vi "Teleop.vi"(10 "Match Info":T2={"Autonomous Elapsed Seconds"=0.0, "TeleOp Elapsed Seconds"=0.0, "Disabled Elapsed Seconds"=0.0, "Visited Autonomous"=FALSE, "Visited TeleOp"=FALSE, "Visited Disabled"=FALSE, "Autonomous Settings"={"Autonomous Style"=enum."Independent", "VI Refnum"=refnum}}, 11 "Call Context":T3) -> ()   [LabVIEW 2019]
doc: "This VI is called for each TeleOp packet received from the DS where the robot is not disabled. It is often used to read from the joysticks and update I/O or to update setpoints for timed control loops. It should complete and return within 20 milliseconds or it may miss DS packets."
uses:
  <vilib>/Rock Robotics/WPI/DriverStation/WPI_DriverStationDerivedRobotMode.ctl
  <vilib>/Rock Robotics/WPI/DriverStation/WPI_DriverStationMatch Info.ctl
  <vilib>/Rock Robotics/WPI/ThirdParty/Phoenix-LabVIEW/Motor Controller/Controls/CTRE_Phoenix_MotorControl_ControlMode.ctl
  <vilib>/Rock Robotics/WPI/Solenoid/WPI_SolenoidValue.ctl
  <vilib>/Rock Robotics/Network Tables/NT Read Boolean.vi
  <vilib>/Rock Robotics/Network Tables/NT Read Number.vi
  <vilib>/Rock Robotics/WPI/Utilities/WPI_GetSetVariantRefNum.vi
  Robot Global Data.vi
  <vilib>/addons/control/pid/pid.llb/PID (DBL).vi
  <vilib>/Rock Robotics/Network Tables/NT Write Number.vi
  <vilib>/Rock Robotics/Network Tables/NT Write Numeric Array.vi
  <vilib>/Rock Robotics/WPI/Solenoid/WPI_SolenoidSetEnum.vi
  <vilib>/addons/control/pid/NI_PID_pid.lvlib
  <vilib>/Rock Robotics/Network Tables/NT Write Boolean.vi
  <vilib>/Rock Robotics/Network Tables/NT Write Boolean Array.vi
  <vilib>/Rock Robotics/Network Tables/NT Write String.vi
panel:
  in  "PID gains":T1={"proportional gain (Kc)"=1.0, "integral time (Ti, min)"=0.01, "derivative time (Td, min)"=0.0} {"derivative time (Td, min)" format="%.3f"; "integral time (Ti, min)" format="%.3f"; "proportional gain (Kc)" format="%.3f"}
  out "Sample Slider 0":dbl(slide) scale=0.0..5.0
  out "Sample Boolean 1":bool
  out "Sample Boolean 0":bool
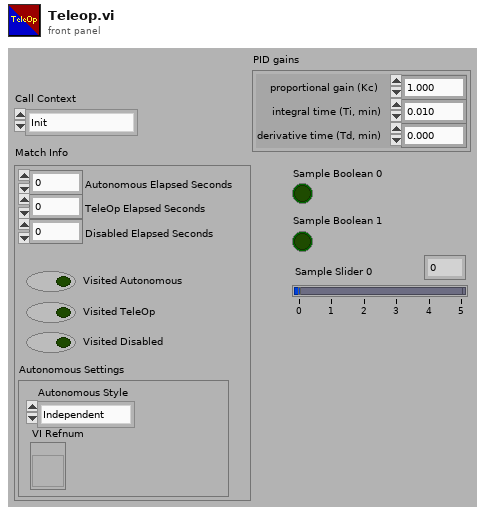
[diagram p1: front panel]
types:
  T1 = cluster{"proportional gain (Kc)":dbl, "integral time (Ti, min)":dbl, "derivative time (Td, min)":dbl}
  T2 = typedef "WPI_DriverStationMatch Info.ctl" = cluster{"Autonomous Elapsed Seconds":dbl, "TeleOp Elapsed Seconds":dbl, "Disabled Elapsed Seconds":dbl, "Visited Autonomous":bool, "Visited TeleOp":bool, "Visited Disabled":bool, "Autonomous Settings":cluster{"Autonomous Style":enum16{"Iterative", "Independent"}, "VI Refnum":refnum<vi>}}
  T3 = typedef "WPI_DriverStationDerivedRobotMode.ctl" = enum16{"Init", "Execute", "Stop"}
  T4 = typedef "CTRE_Phoenix_MotorControl_ControlMode.ctl" = u16
  T5 = typedef "WPI_JoystickDevRef.ctl" = cluster{"Device":T6}
  T6 = typedef "WPI_JoystickDeviceEnum.ctl" = enum16{"USB 0", "USB 1", "USB 2", "USB 3", "USB 4", "USB 5"}
  T7 = typedef "WPI_RobotDriveDevRef.ctl" = cluster{"DevStatus":errorcluster, "Motors[]":T8[], "Square Inputs":bool, "Max Output":dbl}
  T8 = typedef "WPI_MotorControlDeviceRef.ctl" = cluster{"DeviceStatus":errorcluster, "Type":T9, "PWM":cluster{"PWM Channel":T10, "DeadBand":T11}, "CAN":cluster{"Device Number":u8, "SetOutput VI Ref":variant, "GetOutput VI Ref":variant, "Enable VI Ref":variant, "Disable VI Ref":variant, "Data":variant}, "Invert":bool, "DIO PWM":cluster{"PWM \"Enable\" Channel":T10, "DIOChannel":T12, "PWM Rate":dbl}}
  T9 = typedef "WPI_MotorControlType.ctl" = enum16{"PWM", "CAN", "DIO PWM"}
  T10 = typedef "FPGA_DIOPWMChannel.ctl" = enum8{"PWM 0", "PWM 1", "PWM 2", "PWM 3", "PWM 4", "PWM 5", "PWM 6", "PWM 7", "PWM 8", "PWM 9", "PWM MXP 0", "PWM MXP 1", "PWM MXP 2", "PWM MXP 3", "PWM MXP 4", "PWM MXP 5", "PWM MXP 6", "PWM MXP 7", "PWM MXP 8", "PWM MXP 9", "Invalid"}
  T11 = typedef "WPI_PWMDeadband.ctl" = cluster{"Name":string, "maxPositivePwm":i32, "minPositivePwm":i32, "centerPwm":i32, "maxNegativePwm":i32, "minNegativePwm":i32, "angularRange":u16}
  T12 = typedef "FPGA_DIOChannel.ctl" = enum8{"DIO 0", "DIO 1", "DIO 2", "DIO 3", "DIO 4", "DIO 5", "DIO 6", "DIO 7", "DIO 8", "DIO 9", "DIO MXP 0", "DIO MXP 1", "DIO MXP 2", "DIO MXP 3", "DIO MXP 4", "DIO MXP 5", "DIO MXP 6", "DIO MXP 7", "DIO MXP 8", "DIO MXP 9", "DIO MXP 10", "DIO MXP 11", "DIO MXP 12", "DIO MXP 13", "DIO MXP 14", "DIO MXP 15", "SPI Port CS1", "SPI Port CS2", "SPI Port CS3", "SPI Port MISO", "SPI Port MOSI", "Invalid"}
  T13 = cluster{"Buttons[0]":bool, "Buttons[1]":bool, "Buttons[2]":bool, "Buttons[3]":bool, "Buttons[4]":bool, "Buttons[5]":bool, "Buttons[6]":bool, "Buttons[7]":bool, "Buttons[8]":bool, "Buttons[9]":bool}
  T14 = cluster{"Axes[0]":dbl, "Axes[1]":dbl, "Axes[2]":dbl, "Axes[3]":dbl, "Axes[4]":dbl, "Axes[5]":dbl, "Axes[6]":dbl, "Axes[7]":dbl, "Axes[8]":dbl}
  T15 = typedef "WPI_DriverStationAllianceInfo.ctl" = enum16{"Red", "Blue", "Invalid"}
  T16 = typedef "WPI_SolenoidDevRef.ctl" = cluster{"DevStatus":errorcluster, "Pneumatics Control Module":u8, "Forward Solenoid Channel":T17, "Reverse Solenoid Channel":T17}
  T17 = typedef "WPI_SolenoidChannel.ctl" = enum8{"Solenoid 0", "Solenoid 1", "Solenoid 2", "Solenoid 3", "Solenoid 4", "Solenoid 5", "Solenoid 6", "Solenoid 7", "Invalid"}
  T18 = typedef "WPI_SolenoidValue.ctl" = enum16{"Off", "On", "Forward", "Reverse"}
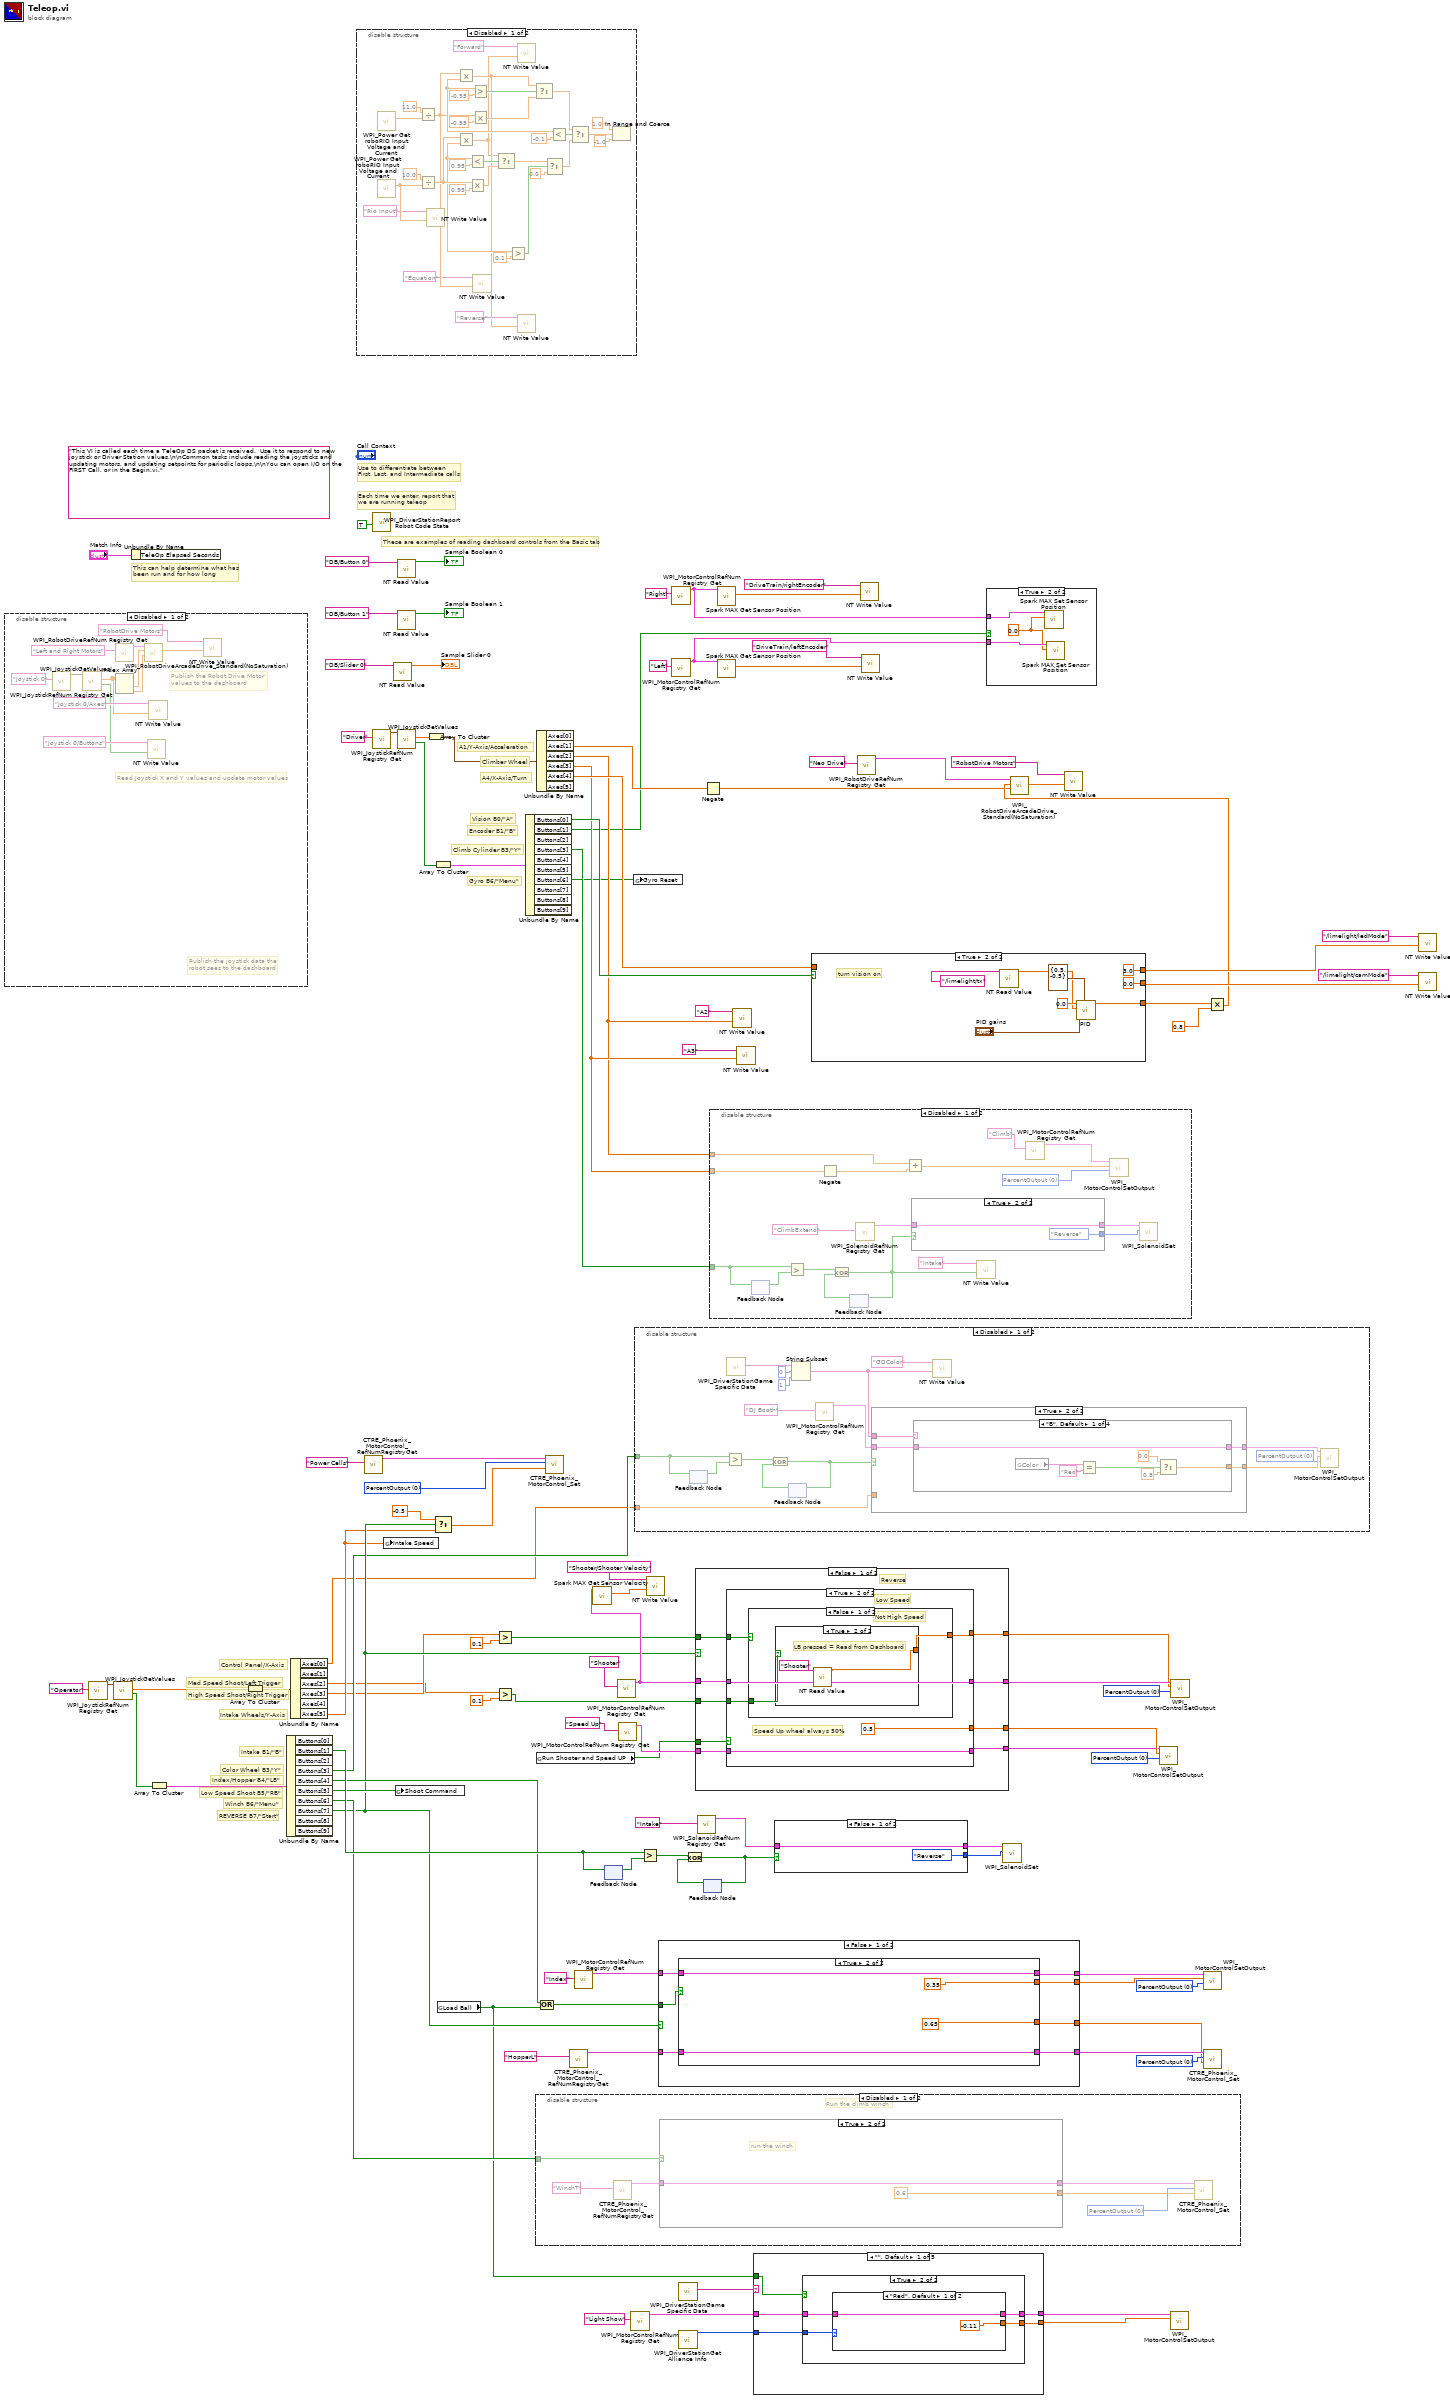
[diagram p0: block diagram]
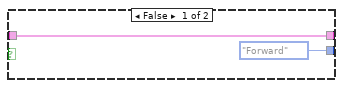
[diagram p2: hidden frame]
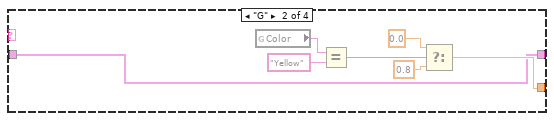
[diagram p5: hidden frame]
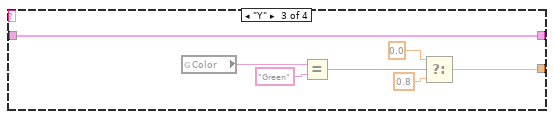
[diagram p6: hidden frame]
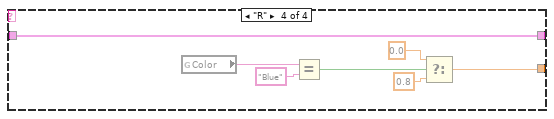
[diagram p7: hidden frame]
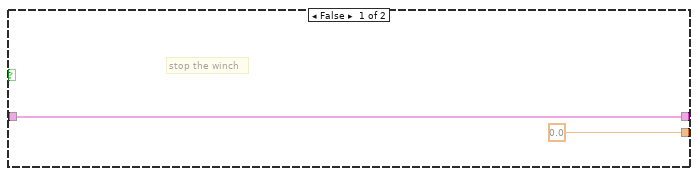
[diagram p9: hidden frame]
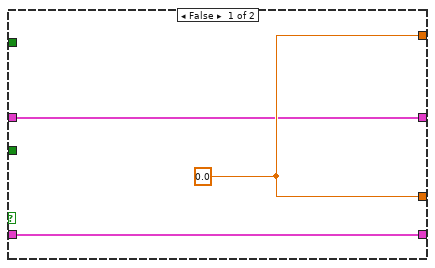
[diagram p12: hidden frame]
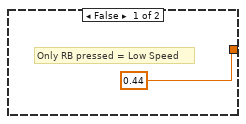
[diagram p13: hidden frame]
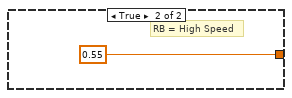
[diagram p14: hidden frame]
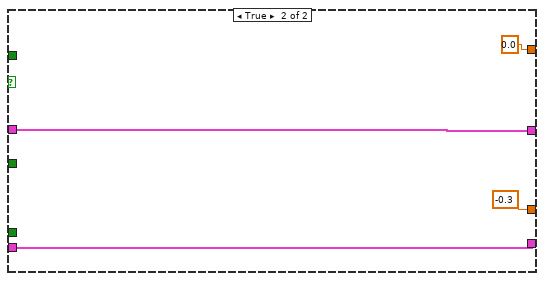
[diagram p15: hidden frame]
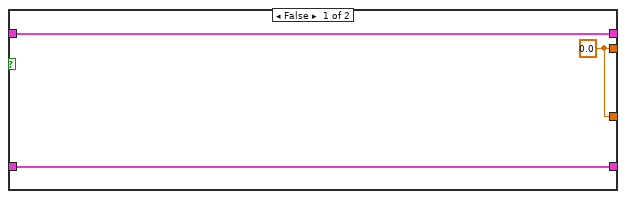
[diagram p16: hidden frame]
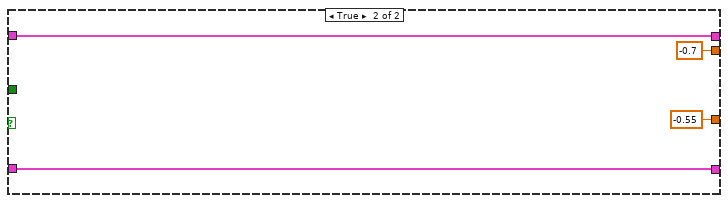
[diagram p17: hidden frame]
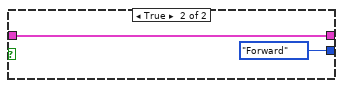
[diagram p18: hidden frame]
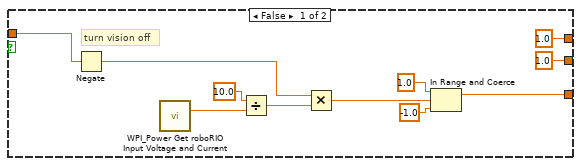
[diagram p20: hidden frame]
diagram:
  w46 = T4 0 items=["PercentOutput"=0, "Position"=1, "Velocity"=2, "Current"=3, "Follower"=5, "MotionProfile"=6, "MotionMagic"=7, "MotionProfileArc"=10, "Disabled"=15] ("Control Mode")
  w49 = T4 0 items=["PercentOutput"=0, "Position"=1, "Velocity"=2, "Current"=3, "Follower"=5, "MotionProfile"=6, "MotionMagic"=7, "MotionProfileArc"=10, "Disabled"=15] ("Control Mode")
  w56 = T4 0 items=["PercentOutput"=0, "Position"=1, "Velocity"=2, "Current"=3, "Follower"=5, "MotionProfile"=6, "MotionMagic"=7, "MotionProfileArc"=10, "Disabled"=15] ("Control Mode")
  w62 = T4 0 items=["PercentOutput"=0, "Position"=1, "Velocity"=2, "Current"=3, "Follower"=5, "MotionProfile"=6, "MotionMagic"=7, "MotionProfileArc"=10, "Disabled"=15] ("Control Mode")
  w64 = T4 0 items=["PercentOutput"=0, "Position"=1, "Velocity"=2, "Current"=3, "Follower"=5, "MotionProfile"=6, "MotionMagic"=7, "MotionProfileArc"=10, "Disabled"=15] ("Control Mode")
  (unwired) "This VI is called each time a TeleOp DS packet is received.  Use it to respond to new joystick or Driver Station values.\n\nCommon tasks include reading the joysticks and updating motors, and updating setpoints for periodic loops.\n\nYou can open I/O on the FIRST Call, or in the Begin.vi."
  # "Med Speed Shoot/Left Trigger"
  # "High Speed Shoot/Right Trigger"
  # "Color Wheel B3/'Y\""
  # "Gyro B6/\"Menu\""
  # "Encoder B1/\"B\""
  # "Climber Wheel"
  # "Climb Cylinder B3/\"Y\""
  # "A1/Y-Axis/Acceleration"
  # "A4/X-Axis/Turn"
  # "Vision B0/\"A\""
  # "Control Panel/X-Axis"
  # "Intake Wheels/Y-Axis"
  # "REVERSE B7/\"Start\""
  # "Winch B6/\"Menu\""
  # "Low Speed Shoot B5/\"RB\""
  # "Index/Hopper B4/\"LB\""
  # "Intake B1/\"B\""
  # "These are examples of reading dashboard controls from the Basic tab"
  # "Each time we enter, report that\nwe are running teleop"
  # "Use to differentiate between\nFirst, Last, and Intermediate calls"
  # "This can help determine what has\nbeen run and for how long"
  n1 = disable-structure shown="Disabled" {
    frame Disabled {
      # "Publish the Robot Drive Motor\nvalues to the dashboard"
      # "Publish the joystick data the\nrobot sees to the dashboard"
      # "Read Joystick X and Y values and update motor values"
      n2 = call <vilib>:"WPI_JoystickRefNum Registry Get.vi"("refnum name"="Joystick 0") -> ("JoystickDevRef"=w116:T5)  [unwired: 1 in, 9 out]
      n3 = call <vilib>:"WPI_JoystickGetValues.vi"("JoystickDevRef"=w116) -> ("Buttons"=w111:bool[], "Axes"=w112:dbl[])  [unwired: 6 in, 3 out]
      n4 = call <vilib>:"WPI_RobotDriveRefNum Registry Get.vi"("refnum name"="Left and Right Motors") -> ("RobotDriveDevRef"=w119:T7)  [unwired: 1 in, 9 out]
      n5 = Index Array(array=w112) -> (element #1=w118:dbl, element #2=w115:dbl)  [unwired: 2 in]
      n6 = call <vilib>:"WPI_RobotDriveArcadeDrive_Standard(NoSaturation).vi"("Y axis value"=w115, "X axis value"=w118, "RobotDriveDevRef"=w119) -> ("Motor Values"=w110:dbl[])  [unwired: 1 in, 7 out]
      n7 = call-poly <vilib>:"NT Write Value.vi"("Boolean Array"=w111, "Name"="Joystick 0/Buttons") -> ()  [unwired: 9 in, 1 out]
      n8 = call-poly <vilib>:"NT Write Value.vi"("Numeric Array"=w112, "Name"="Joystick 0/Axes") -> ()  [unwired: 9 in, 1 out]
      n9 = call-poly <vilib>:"NT Write Value.vi"("Numeric Array"=w110, "Name"="RobotDrive Motors") -> ()  [unwired: 9 in, 1 out]
    }
    frame Enabled {
    }
  }
  n10 = call <vilib>:"WPI_JoystickRefNum Registry Get.vi"("refnum name"="Operator") -> ("JoystickDevRef"=w75:T5)  [unwired: 9 in, 1 out]
  n11 = call <vilib>:"WPI_JoystickGetValues.vi"("JoystickDevRef"=w75) -> ("Buttons"=w48:bool[], "Axes"=w79:dbl[])  [unwired: 6 in, 3 out]
  n12 = Unbundle By Name("Match Info") -> ()  [unwired: 1 out]
  n13 = Array To Cluster(array=w48) -> (cluster=w77:T13)
  n14 = Array To Cluster(array=w79) -> (cluster=w78:T14)
  n15 = Unbundle By Name(w77) -> ("Buttons[1]"=w42:bool, "Buttons[3]"=w10:bool, "Buttons[4]"=w41:bool, "Buttons[5]"=w38:bool, "Buttons[6]"=w37:bool, "Buttons[7]"=w30:bool)  [unwired: 4 out]
  n16 = Unbundle By Name(w78) -> ("Axes[0]"=w9:dbl, "Axes[2]"=w1:dbl, "Axes[3]"=w5:dbl, "Axes[5]"=w28:dbl)  [unwired: 2 out]
  n17 = disable-structure shown="Disabled" {
    frame Disabled {
      n18 = call <vilib>:"WPI_Power Get roboRIO Input Voltage and Current.vi"() -> ("roboRIO input voltage (V)"=w148:dbl)  [unwired: 13 in, 2 out]
      n19 = call <vilib>:"WPI_Power Get roboRIO Input Voltage and Current.vi"() -> ("roboRIO input voltage (V)"=w129:dbl)  [unwired: 13 in, 2 out]
      n20 = Divide(x=11.0, y=w148) -> (x/y=w122:dbl)
      n21 = Divide(x=10.0, y=w129) -> (x/y=w132:dbl)
      n22 = call-poly <vilib>:"NT Write Value.vi"("Numeric"=w129, "Name"="Rio Input") -> ()  [unwired: 9 in, 1 out]
      n23 = Multiply(x=w132, y=0.95 ("f")) -> (x*y=w134:dbl)
      n24 = Multiply(x=w122, y=-0.95 ("f")) -> (x*y=w142:dbl)
      n25 = call-poly <vilib>:"NT Write Value.vi"("Numeric"=w122, "Name"="Equation") -> ()  [unwired: 9 in, 1 out]
      n26 = Greater?(y=0.1) -> (x=w127:dbl, 0:w151:bool)
      n27 = Multiply(x=w132, y=w127) -> (x*y=w123:dbl)
      n28 = Less?(x=w127, y=0.95) -> (x < y?=w136:bool)
      n29 = Select(t=w123, s=w136, f=w134) -> (s? t:f=w133:dbl)
      n30 = call-poly <vilib>:"NT Write Value.vi"("Numeric"=w123, "Name"="Forward") -> ()  [unwired: 9 in, 1 out]
      n31 = Select(t=w133, s=w151, f=0.0) -> (s? t:f=w125:dbl)
      n32 = Less?(y=-0.1) -> (x=w126:dbl, x < y?=w149:bool)
      n33 = Multiply(x=w122, y=w126) -> (x*y=w124:dbl)
      n34 = Greater?(x=w126, y=-0.95) -> (0:w145:bool)
      n35 = call-poly <vilib>:"NT Write Value.vi"("Numeric"=w124, "Name"="Reverse") -> ()  [unwired: 9 in, 1 out]
      n36 = Select(t=w124, s=w145, f=w142) -> (s? t:f=w144:dbl)
      n37 = Select(t=w144, s=w149, f=w125) -> (s? t:f=w141:dbl)
      n38 = In Range and Coerce(upper limit=1.0, x=w141, lower limit=-1.0) -> ()  [unwired: 2 out]
    }
    frame Enabled {
    }
  }
  n39 = call <vilib>:"CTRE_Phoenix_MotorControl_RefNumRegistryGet.vi"("refnum name"="Power Cells") -> ("PhoenixMotorControlDevRef"=w65:T8)  [unwired: 9 in, 1 out]
  n40 = call <vilib>:"WPI_DriverStationReport Robot Code State.vi"("TeleOp"=TRUE ("Autonomous")) -> ()  [unwired: 10 in, 1 out]
  n41 = call <vilib>:"WPI_JoystickRefNum Registry Get.vi"("refnum name"="Driver") -> ("JoystickDevRef"=w95:T5)  [unwired: 9 in, 1 out]
  n42 = global write "Robot Global Data.vi" "Intake Speed"(w28) -> ()
  n43 = call-poly <vilib>:"NT Read Value.vi"("Name"="DB/Slider 0" ("refnum name")) -> ("Numeric"=→"Sample Slider 0":dbl)  [unwired: 9 in, 1 out]
  n44 = global write "Robot Global Data.vi" "Shoot Command"(w38) -> ()
  n45 = call-poly <vilib>:"NT Read Value.vi"("Name"="DB/Button 0" ("refnum name")) -> ("Boolean"=→"Sample Boolean 0":bool)  [unwired: 9 in, 1 out]
  n46 = call-poly <vilib>:"NT Read Value.vi"("Name"="DB/Button 1" ("refnum name")) -> ("Boolean"=→"Sample Boolean 1":bool)  [unwired: 9 in, 1 out]
  n47 = call <vilib>:"WPI_JoystickGetValues.vi"("JoystickDevRef"=w95) -> ("Buttons"=w98:bool[], "Axes"=w100:dbl[])  [unwired: 6 in, 3 out]
  n48 = Array To Cluster(array=w100) -> (cluster=w99:T14)
  n49 = Array To Cluster(array=w98) -> (cluster=w97:T13)
  n50 = Select(t=-0.5, s=w30, f=w28) -> (s? t:f=w29:dbl)
  n51 = global read "Robot Global Data.vi" "Load Ball"() -> (w8:bool)
  n52 = Greater?(x=w5, y=0.1) -> (0:w6:bool)
  n53 = Greater?(x=w1, y=0.1) -> (0:w2:bool)
  n54 = Unbundle By Name(w97) -> ("Buttons[0]"=w81:bool, "Buttons[1]"=w16:bool, "Buttons[3]"=w33:bool, "Buttons[6]"=w26:bool)  [unwired: 6 out]
  n55 = disable-structure shown="Disabled" {
    disable-tunnel: w37 -> [w159 _]
    frame Disabled {
      w155 = T4 0 items=["PercentOutput"=0, "Position"=1, "Velocity"=2, "Current"=3, "Follower"=5, "MotionProfile"=6, "MotionMagic"=7, "MotionProfileArc"=10, "Disabled"=15] ("Control Mode")
      # "Run the climb winch"
      n56 = call <vilib>:"CTRE_Phoenix_MotorControl_RefNumRegistryGet.vi"("refnum name"="WinchT") -> ("PhoenixMotorControlDevRef"=w156:T8)  [unwired: 9 in, 1 out]
      n57 = case shown="True" w159 {
        tunnel: [w161 w163] -> w157
        tunnel: w156 -> [w161 w163]
        tunnel: [0.0 ("Output") 0.6 ("Output")] -> w154
        frame False {
          # "stop the winch"
        }
        frame True {
          # "run the winch"
        }
      }
      n58 = call <vilib>:"CTRE_Phoenix_MotorControl_Set.vi"("Output"=w154, "Control Mode"=w155, "PhoenixMotorControlDevRef"=w157) -> ()  [unwired: 7 in, 2 out]
    }
    frame Enabled {
    }
  }
  n59 = global read "Robot Global Data.vi" "Run Shooter and Speed UP"() -> (w39:bool)
  n60 = Unbundle By Name(w99) -> ("Axes[1]"=w82:dbl, "Axes[2]"=w31:dbl, "Axes[3]"=w32:dbl, "Axes[4]"=w80:dbl)  [unwired: 2 out]
  n61 = Or(x=w41, y=w8) -> (x .or. y?=w40:bool)
  n62 = call <vilib>:"CTRE_Phoenix_MotorControl_Set.vi"("Output"=w29, "Control Mode"=w64, "PhoenixMotorControlDevRef"=w65) -> ()  [unwired: 7 in, 2 out]
  n63 = call <vilib>:"CTRE_Phoenix_MotorControl_RefNumRegistryGet.vi"("refnum name"="HopperL") -> ("PhoenixMotorControlDevRef"=w61:T8)  [unwired: 9 in, 1 out]
  n64 = call <vilib>:"WPI_MotorControlRefNum Registry Get.vi"("refnum name"="Index") -> ("MotorControlDevRef"=w53:T8)  [unwired: 9 in, 1 out]
  n65 = feedback #1() -> (w72:bool)  [unwired: 1 in]
  n66 = feedback-in #1(w42) -> ()
  n67 = call <vilib>:"WPI_MotorControlRefNum Registry Get.vi"("refnum name"="Shooter") -> ("MotorControlDevRef"=w44:T8)  [unwired: 9 in, 1 out]
  n68 = call <vilib>:"Spark MAX Get Sensor Velocity.vi"("MotorControlDevRef in"=w44) -> ("Sensor Velocity"=w12:dbl)  [unwired: 7 in, 3 out]
  n69 = call <vilib>:"WPI_MotorControlRefNum Registry Get.vi"("refnum name"="Speed Up") -> ("MotorControlDevRef"=w55:T8)  [unwired: 9 in, 1 out]
  n70 = call <vilib>:"WPI_MotorControlRefNum Registry Get.vi"("refnum name"="Light Show") -> ("MotorControlDevRef"=w92:T8)  [unwired: 9 in, 1 out]
  n71 = global write "Robot Global Data.vi" "Gyro Reset"(w26) -> ()
  n72 = disable-structure shown="Disabled" {
    disable-tunnel: w10 -> [w165 _]
    disable-tunnel: w9 -> [w164 _]
    frame Disabled {
      w175 = T4 0 items=["PercentOutput"=0, "Position"=1, "Velocity"=2, "Current"=3, "Follower"=5, "MotionProfile"=6, "MotionMagic"=7, "MotionProfileArc"=10, "Disabled"=15] ("Control Mode")
      n73 = feedback #2() -> (w167:bool)  [unwired: 1 in]
      n74 = feedback-in #2(w165) -> ()
      n75 = Greater?(x=w165, y=w167) -> (0:w168:bool)
      n76 = call <vilib>:"WPI_DriverStationGame Specific Data.vi"() -> ("Game Specific Data"=w174:string)  [unwired: 11 in]
      n77 = feedback #3() -> (w169:bool)  [unwired: 1 in]
      n78 = Exclusive Or(1:w169, 2:w168) -> (0:w166:bool)
      n79 = feedback-in #3(w166) -> ()
      n80 = String Subset(string=w174, offset (0)=0, length (rest)=1 ("length (rest)")) -> (substring=w171:string)
      n81 = call <vilib>:"WPI_MotorControlRefNum Registry Get.vi"("refnum name"="DJ Booth") -> ("MotorControlDevRef"=w178:T8)  [unwired: 9 in, 1 out]
      n82 = case shown="True" w166 {
        tunnel: w178 -> [w181 w185]
        tunnel: [w180 w184] -> w177
        tunnel: [w181 w183] -> w176
        tunnel: w171 -> [_ w182]
        tunnel: w164 -> [w180 _]
        frame False {
        }
        frame True {
          n83 = case shown="\"B\", Default" w182 {
            tunnel: w185 -> [w191 w193 w200 w207]
            tunnel: [w191 w193 w200 w207] -> w183
            tunnel: [w192 w194 w201 w208] -> w184
            frame "B", Default {
              n84 = global read "Robot Global Data.vi" "Color"() -> (w190:string)
              n85 = Equal?(x=w190, y="Red") -> (x = y?=w188:bool)
              n86 = Select(t=0.0, s=w188, f=0.8) -> (s? t:f=w192:dbl)
            }
            frame "G" {
              n87 = global read "Robot Global Data.vi" "Color"() -> (w198:string)
              n88 = Equal?(x=w198, y="Yellow") -> (x = y?=w199:bool)
              n89 = Select(t=0.0, s=w199, f=0.8) -> (s? t:f=w194:dbl)
            }
            frame "Y" {
              n90 = global read "Robot Global Data.vi" "Color"() -> (w205:string)
              n91 = Equal?(x=w205, y="Green") -> (x = y?=w206:bool)
              n92 = Select(t=0.0, s=w206, f=0.8) -> (s? t:f=w201:dbl)
            }
            frame "R" {
              n93 = global read "Robot Global Data.vi" "Color"() -> (w213:string)
              n94 = Equal?(x=w213, y="Blue") -> (x = y?=w211:bool)
              n95 = Select(t=0.0, s=w211, f=0.8) -> (s? t:f=w208:dbl)
            }
          }
        }
      }
      n96 = call-poly <vilib>:"NT Write Value.vi"("String"=w171, "Name"="GDColor") -> ()  [unwired: 9 in, 1 out]
      n97 = call <vilib>:"WPI_MotorControlSetOutput.vi"("options"=w175, "Output"=w177, "MotorControlDevRef"=w176) -> ()  [unwired: 6 in, 3 out]
    }
    frame Enabled {
    }
  }
  n98 = Greater?(x=w42, y=w72) -> (0:w73:bool)
  n99 = call-poly <vilib>:"NT Write Value.vi"("Numeric"=w12, "Name"="Shooter/Shooter Velocity") -> ()  [unwired: 9 in, 1 out]
  n100 = case shown="False" w30 {
    tunnel: w61 -> [w220 w230]
    tunnel: [w219 w230] -> w60
    tunnel: [w218 -0.55 ("Numeric")] -> w59
    tunnel: w53 -> [w217 w231]
    tunnel: [w216 w231] -> w51
    tunnel: [w215 -0.7 ("Numeric")] -> w50
    tunnel: w40 -> [w214 _]
    frame False {
      n101 = case shown="True" w214 {
        tunnel: w217 -> [w223 w227]
        tunnel: [w223 w227] -> w216
        tunnel: [w221 0.35 ("Output")] -> w215
        tunnel: w220 -> [w222 w226]
        tunnel: [w222 w226] -> w219
        tunnel: [w221 0.65 ("Output")] -> w218
        frame False {
          w221 = 0.0 ("Output")
        }
        frame True {
        }
      }
    }
    frame True {
    }
  }
  n102 = call <vilib>:"WPI_MotorControlRefNum Registry Get.vi"("refnum name"="Right") -> ("MotorControlDevRef"=w18:T8)  [unwired: 9 in, 1 out]
  n103 = call <vilib>:"WPI_MotorControlRefNum Registry Get.vi"("refnum name"="Left") -> ("MotorControlDevRef"=w17:T8)  [unwired: 9 in, 1 out]
  n104 = call <vilib>:"WPI_DriverStationGame Specific Data.vi"() -> ("Game Specific Data"=w94:string)  [unwired: 11 in]
  n105 = call <vilib>:"WPI_DriverStationGet Alliance Info.vi"() -> ("Alliance"=w25:T15)  [unwired: 6 in, 5 out]
  n106 = case shown="False" w30 {
    tunnel: [w233 -0.3 ("Numeric")] -> w57
    tunnel: w55 -> [w240 w259]
    tunnel: [w239 w259] -> w54
    tunnel: [w238 w256] -> w45
    tunnel: w44 -> [w237 w256]
    tunnel: [w236 0.0 ("Numeric")] -> w43
    tunnel: w39 -> [w235 _]
    tunnel: w6 -> [w234 _]
    tunnel: w2 -> [w232 _]
    frame False {
      # "Reverse"
      n107 = case shown="True" w235 {
        tunnel: [w242 0.5 ("Numeric")] -> w233
        tunnel: w240 -> [w243 w249]
        tunnel: [w243 w249] -> w239
        tunnel: [w241 w248] -> w238
        tunnel: w237 -> [w241 w248]
        tunnel: [w242 w246] -> w236
        tunnel: w234 -> [_ w245]
        tunnel: w232 -> [_ w244]
        frame False {
          w242 = 0.0 ("Numeric")
        }
        frame True {
          # "Low Speed"
          # "Speed Up wheel always 50%"
          n108 = case shown="False" w245 {
            tunnel: [w251 0.55 ("Numeric")] -> w246
            tunnel: w244 -> [w250 _]
            frame False {
              # "Not High Speed"
              n109 = case shown="True" w250 {
                tunnel: [0.44 ("Numeric") w253] -> w251
                frame False {
                  # "Only RB pressed = Low Speed"
                }
                frame True {
                  # "LB pressed = Read from Dashboard"
                  n110 = call-poly <vilib>:"NT Read Value.vi"("Name"="Shooter") -> ("Numeric"=w253:dbl)  [unwired: 9 in, 1 out]
                }
              }
            }
            frame True {
              # "RB = High Speed"
            }
          }
        }
      }
    }
    frame True {
    }
  }
  n111 = call <vilib>:"WPI_SolenoidRefNum Registry Get.vi"("refnum name"="Intake") -> ("SolenoidDevRef"=w69:T16)  [unwired: 9 in, 1 out]
  n112 = feedback #4() -> (w74:bool)  [unwired: 1 in]
  n113 = Exclusive Or(1:w74, 2:w73) -> (0:w67:bool)
  n114 = feedback-in #4(w67) -> ()
  n115 = Negate(x=w82) -> (-x=w7:dbl)
  n116 = disable-structure shown="Disabled" {
    disable-tunnel: w33 -> [w266 _]
    disable-tunnel: w32 -> [w265 _]
    disable-tunnel: w31 -> [w263 _]
    frame Disabled {
      w260 = T4 0 items=["PercentOutput"=0, "Position"=1, "Velocity"=2, "Current"=3, "Follower"=5, "MotionProfile"=6, "MotionMagic"=7, "MotionProfileArc"=10, "Disabled"=15] ("Control Mode")
      n117 = feedback #5() -> (w273:bool)  [unwired: 1 in]
      n118 = feedback-in #5(w266) -> ()
      n119 = Greater?(x=w266, y=w273) -> (0:w274:bool)
      n120 = Negate(x=w265) -> (-x=w262:dbl)
      n121 = feedback #6() -> (w275:bool)  [unwired: 1 in]
      n122 = Exclusive Or(1:w275, 2:w274) -> (0:w268:bool)
      n123 = feedback-in #6(w268) -> ()
      n124 = call <vilib>:"WPI_SolenoidRefNum Registry Get.vi"("refnum name"="ClimbExtend") -> ("SolenoidDevRef"=w270:T16)  [unwired: 9 in, 1 out]
      n125 = Add(x=w263, y=w262) -> (x+y=w261:dbl)
      n126 = case shown="True" w268 {
        tunnel: [WPI_SolenoidValue."Forward" ("Value") WPI_SolenoidValue."Reverse" ("Value")] -> w271
        tunnel: w270 -> [w278 w279]
        tunnel: [w278 w279] -> w269
        frame False {
        }
        frame True {
        }
      }
      n127 = call-poly <vilib>:"NT Write Value.vi"("Boolean"=w268, "Name"="Intake") -> ()  [unwired: 9 in, 1 out]
      n128 = call <vilib>:"WPI_MotorControlRefNum Registry Get.vi"("refnum name"="Climb") -> ("MotorControlDevRef"=w264:T8)  [unwired: 9 in, 1 out]
      n129 = call <vilib>:"WPI_MotorControlSetOutput.vi"("options"=w260, "Output"=w261, "MotorControlDevRef"=w264) -> ()  [unwired: 6 in, 3 out]
      n130 = call-poly <vilib>:"WPI_SolenoidSet.vi"("Value"=w271, "SolenoidDevRef"=w269) -> ()  [unwired: 8 in, 2 out]
    }
    frame Enabled {
    }
  }
  n131 = call <vilib>:"Spark MAX Get Sensor Position.vi"("MotorControlDevRef in"=w18) -> ("Sensor Position"=w23:dbl)  [unwired: 7 in, 3 out]
  n132 = call <vilib>:"Spark MAX Get Sensor Position.vi"("MotorControlDevRef in"=w17) -> ("Sensor Position"=w21:dbl)  [unwired: 7 in, 3 out]
  n133 = call-poly <vilib>:"NT Write Value.vi"("Numeric"=w31, "Name"="A2") -> ()  [unwired: 9 in, 1 out]
  n134 = call-poly <vilib>:"NT Write Value.vi"("Numeric"=w32, "Name"="A3") -> ()  [unwired: 9 in, 1 out]
  n135 = case shown="\"\", Default" w94 {
    tunnel: w92 -> [w285 w303 w304 w306 w308]
    tunnel: [w284 w303 w304 w306 w308] -> w91
    tunnel: [w283 0.87 ("Output") 0.61 ("Output") 0.77 ("Output") 0.69 ("Output")] -> w90
    tunnel: w25 -> [w282 _ _ _ _]
    tunnel: w8 -> [w281 _ _ _ _]
    frame "", Default {
      n136 = case shown="True" w281 {
        tunnel: w285 -> [w289 w296]
        tunnel: [w288 w295] -> w284
        tunnel: [w287 w294] -> w283
        tunnel: w282 -> [w286 w297]
        frame False {
          n137 = case shown="\"Blue\", Default" w286 {
            tunnel: w289 -> [w291 w293]
            tunnel: [w291 w293] -> w288
            tunnel: [-0.29 ("Output") -0.31 ("Output")] -> w287
            frame "Blue", Default {
            }
            frame "Red" {
            }
          }
        }
        frame True {
          n138 = case shown="\"Red\", Default" w297 {
            tunnel: w296 -> [w299 w301]
            tunnel: [w299 w301] -> w295
            tunnel: [-0.11 ("Output") -0.09 ("Output")] -> w294
            frame "Red", Default {
            }
            frame "Blue" {
            }
          }
        }
      }
    }
    frame "B" {
    }
    frame "R" {
    }
    frame "G" {
    }
    frame "Y" {
    }
  }
  n139 = case shown="False" w67 {
    tunnel: [WPI_SolenoidValue."Reverse" ("Value") WPI_SolenoidValue."Forward" ("Value")] -> w70
    tunnel: w69 -> [w310 w313]
    tunnel: [w310 w313] -> w68
    frame False {
    }
    frame True {
    }
  }
  n140 = case shown="True" w81 {
    tunnel: [w319 w328] -> w14
    tunnel: [1.0 ("Numeric") 3.0 ("Numeric")] -> w85
    tunnel: [1.0 ("Numeric") 0.0 ("Numeric")] -> w83
    tunnel: w80 -> [w315 _]
    frame False {
      # "turn vision off"
      n141 = Negate(x=w315) -> (-x=w314:dbl)
      n142 = call <vilib>:"WPI_Power Get roboRIO Input Voltage and Current.vi"() -> ("roboRIO input voltage (V)"=w322:dbl)  [unwired: 13 in, 2 out]
      n143 = Divide(x=10.0, y=w322) -> (x/y=w316:dbl)
      n144 = Multiply(x=w314, y=w316) -> (x*y=w320:dbl)
      n145 = In Range and Coerce(upper limit=1.0, x=w320, lower limit=-1.0) -> (coerced(x)=w319:dbl)  [unwired: 1 out]
    }
    frame True {
      # "turn vision on"
      n146 = call-poly <vilib>:"NT Read Value.vi"("Name"="/limelight/tx") -> ("Numeric"=w330:dbl)  [unwired: 9 in, 1 out]
      n147 = call-poly <vilib>:"PID.vi"("output range"=cluster{"output high":dbl, "output low":dbl} {"output high"=0.5, "output low"=-0.5}, "PID gains"="PID gains", "process variable"=w330, "setpoint"=0.0) -> ("output"=w328:dbl)  [unwired: 6 in, 1 out]
    }
  }
  n148 = call <vilib>:"WPI_RobotDriveRefNum Registry Get.vi"("refnum name"="Neo Drive") -> ("RobotDriveDevRef"=w87:T7)  [unwired: 9 in, 1 out]
  n149 = call-poly <vilib>:"NT Write Value.vi"("Numeric"=w23, "Name"="DriveTrain/rightEncoder") -> ()  [unwired: 9 in, 1 out]
  n150 = call-poly <vilib>:"NT Write Value.vi"("Numeric"=w21, "Name"="DriveTrain/leftEncoder") -> ()  [unwired: 9 in, 1 out]
  n151 = case shown="True" w16 {
    tunnel: w18 -> [_ w335]
    tunnel: w17 -> [_ w334]
    frame False {
    }
    frame True {
      w333 = 0.0 ("Position")
      n152 = call <vilib>:"Spark MAX Set Sensor Position.vi"("Position"=w333, "MotorControlDeviceRef"=w335) -> ()  [unwired: 8 in, 2 out]
      n153 = call <vilib>:"Spark MAX Set Sensor Position.vi"("Position"=w333, "MotorControlDeviceRef"=w334) -> ()  [unwired: 8 in, 2 out]
    }
  }
  n154 = call-poly <vilib>:"WPI_SolenoidSet.vi"("Value"=w70, "SolenoidDevRef"=w68) -> ()  [unwired: 8 in, 2 out]
  n155 = call <vilib>:"WPI_MotorControlSetOutput.vi"("options"=w56, "Output"=w57, "MotorControlDevRef"=w54) -> ()  [unwired: 6 in, 3 out]
  n156 = call <vilib>:"WPI_MotorControlSetOutput.vi"("Output"=w90, "MotorControlDevRef"=w91) -> ()  [unwired: 7 in, 3 out]
  n157 = call <vilib>:"WPI_MotorControlSetOutput.vi"("options"=w46, "Output"=w43, "MotorControlDevRef"=w45) -> ()  [unwired: 6 in, 3 out]
  n158 = call <vilib>:"WPI_MotorControlSetOutput.vi"("options"=w49, "Output"=w50, "MotorControlDevRef"=w51) -> ()  [unwired: 6 in, 3 out]
  n159 = call <vilib>:"CTRE_Phoenix_MotorControl_Set.vi"("Output"=w59, "Control Mode"=w62, "PhoenixMotorControlDevRef"=w60) -> ()  [unwired: 7 in, 2 out]
  n160 = Multiply(x=w14, y=0.8) -> (x*y=w15:dbl)
  n161 = call <vilib>:"WPI_RobotDriveArcadeDrive_Standard(NoSaturation).vi"("Y axis value"=w7, "X axis value"=w15, "RobotDriveDevRef"=w87) -> ("Motor Values"=w89:dbl[])  [unwired: 1 in, 7 out]
  n162 = call-poly <vilib>:"NT Write Value.vi"("Numeric Array"=w89, "Name"="RobotDrive Motors") -> ()  [unwired: 9 in, 1 out]
  n163 = call-poly <vilib>:"NT Write Value.vi"("Numeric"=w85, "Name"="/limelight/ledMode") -> ()  [unwired: 9 in, 1 out]
  n164 = call-poly <vilib>:"NT Write Value.vi"("Numeric"=w83, "Name"="/limelight/camMode") -> ()  [unwired: 9 in, 1 out]
